vi "Test.vi"() -> ()   [LabVIEW 2023]
uses:
  <vilib>/Instr/_visa.llb/VISA Configure Serial Port (Instr).vi
panel:
  in  "Termination Character":u8=10 format="%.0x"
  out "read buffer":string
  in  "error in (no error)":errorcluster
  in  "VISA resource name":refnum<visa-resource-name>
  out "error out":errorcluster
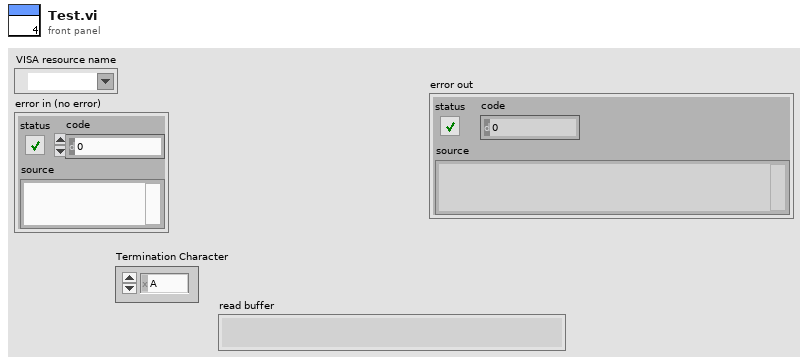
[diagram p1: front panel]
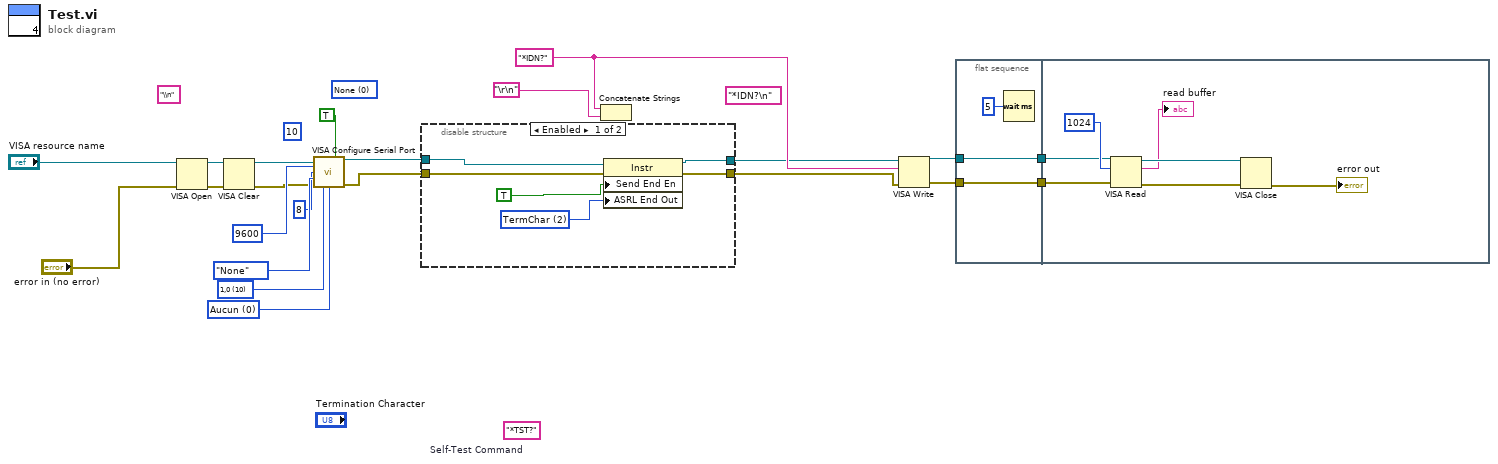
[diagram p0: block diagram]
diagram:
  (unwired) u8 10 ("termination char\n(0xA = '\\n' = LF)")
  (unwired) u16 0 items=["None", "LastBit", "TermChar", "Break"] ("Serial Settings:Serial End Mode for Writes")
  (unwired) "*IDN?\n" ("Command")
  (unwired) "\\n" ("string")
  w14 = u16 0 items=["Aucun", "XON/XOFF", "RTS/CTS", "XON/XOFF & RTS/CTS", "DTR/DSR", "XON/XOFF & DTR/DSR"] ("flow control (0:none)")
  w13 = u16 10 items=["1,0"=10, "1,5"=15, "2,0"=20] ("stop bits (10: 1 bit)")
  (unwired) "*TST?"  # Self-Test Command
  w6 = "*IDN?" ("write buffer")
  n1 = VISA Open(error in (no error)="error in (no error)", VISA resource name="VISA resource name") -> (VISA resource name=w18:refnum<visa-resource-name>, error out=w17:errorcluster)  [unwired: 3 in]
  n2 = VISA Clear(VISA resource name=w18, error in (no error)=w17) -> (VISA resource name out=w9:refnum<visa-resource-name>, error out=w8:errorcluster)
  n3 = call-poly "VISA Configure Serial Port"("VISA resource name"=w9, "Enable Termination\nChar (T)"=TRUE ("Enable Termination\nChar (T)"), "baud rate (9600)"=u32 9600, "data bits (8)"=u16 8, "parity (0:none)"=enum16{"None", "Odd", "Even", "Mark", "Space"}."None", "error in (no error)"=w8, "stop bits (10: 1 bit)"=w13, "flow control (0:none)"=w14) -> ("VISA resource name out"=w5:refnum<visa-resource-name>, "error out"=w4:errorcluster)  [unwired: 6 in]
  n4 = disable-structure shown="Enabled" {
    disable-tunnel: w5 -> [w28 w30]
    disable-tunnel: w4 -> [w27 w29]
    disable-tunnel: [w26 w30] -> w3
    disable-tunnel: [w25 w29] -> w2
    frame Enabled {
      w23 = u16 2 items=["None", "Last Bit", "TermChar", "Break"] ("Serial Settings:End Mode for Writes")
      n5 = property class="Instr"(reference=w28, error in=w27, "Send End En"=TRUE ("Message Based Settings:Send End Enable"), "ASRL End Out"=w23) -> (reference out=w26:refnum<visa-resource-name>, error out=w25:errorcluster)
    }
    frame Disabled {
    }
  }
  n6 = Concatenate Strings(w6, "\r\n") -> ()  [unwired: 1 out]
  n7 = VISA Write(VISA resource name=w3, write buffer=w6, error in (no error)=w2) -> (VISA resource name out=w19:refnum<visa-resource-name>, error out=w20:errorcluster)  [unwired: 1 out]
  n8 = flat-sequence {
    tunnel: w19 -> [w32]
    tunnel: w20 -> [w33]
    tunnel: [w33] -> w16
    tunnel: [w32] -> w15
    tunnel: w16 -> [w36]
    tunnel: w15 -> [w35]
    frame #0 {
      n9 = Wait (ms)(milliseconds to wait=u32 5) -> ()  [unwired: 1 out]
    }
    frame #1 {
      n10 = VISA Read(VISA resource name=w35, byte count=u32 1024, error in (no error)=w36) -> (VISA resource name out=w39:refnum<visa-resource-name>, read buffer=→"read buffer":string, error out=w40:errorcluster)  [unwired: 1 out]
      n11 = VISA Close(VISA resource name=w39, error in (no error)=w40) -> (error out=→"error out":errorcluster)
    }
  }
